vi "0036-Sub_WriteI2C.vi"(0 "device":T2, 1 "書き込み":u8[](array[numeric])=[2], 2 "numBytesToWrite":u8=1, 3 "error out":errorcluster) -> (7 "device 2":T2, 8 "数値":dbl, 10 "error out 2":errorcluster caption="error out")   [LabVIEW 2014]
uses:
  <userlib>/LV-CP2112_2014/LVProject/private/CP2112_device.ctl
  <userlib>/LV-CP2112_2014/LVProject/private/CP2112_SMBUS_S0.ctl
panel:
  out "numByteRead":u8
  out "HID_SMBUS_S0":T1
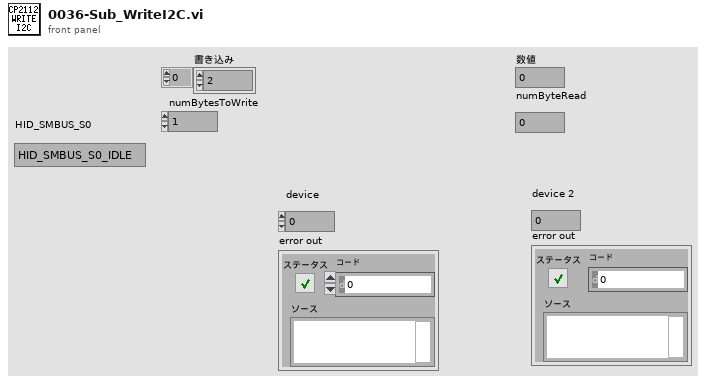
[diagram p1: front panel]
types:
  T1 = typedef "CP2112_SMBUS_S0.ctl" = enum8{"HID_SMBUS_S0_IDLE", "HID_SMBUS_S0_BUSY", "HID_SMBUS_S0_COMPLETE", "HID_SMBUS_S0_ERROR"}
  T2 = typedef "CP2112_device.ctl" = i32
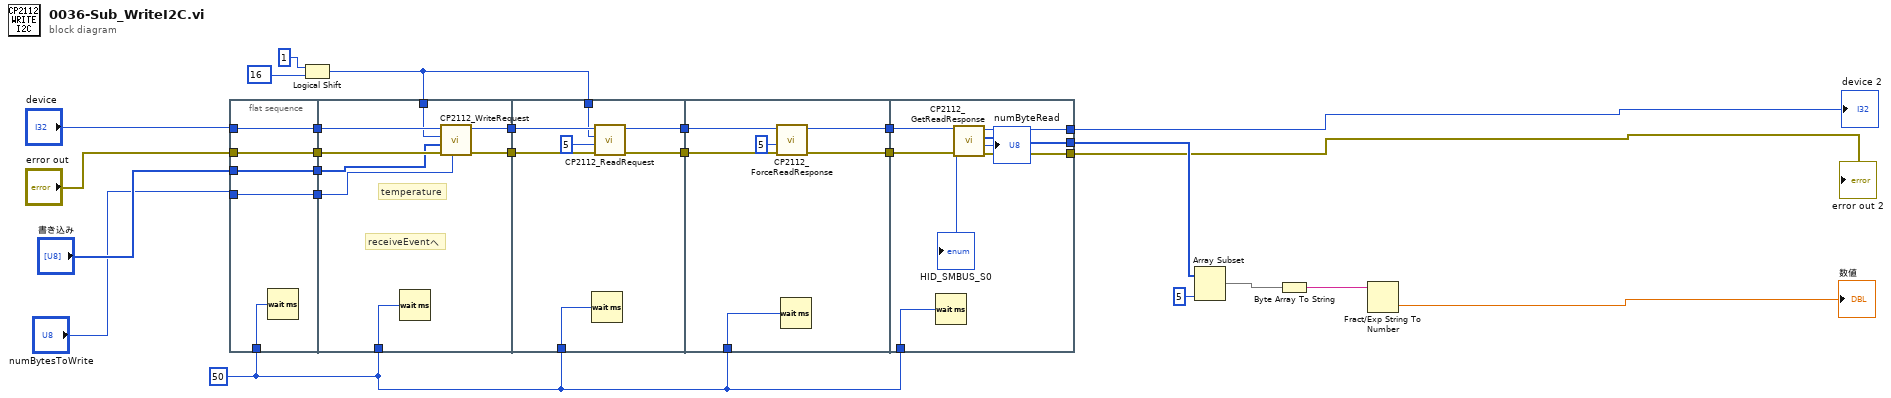
[diagram p0: block diagram]
diagram:
  w1 = u32 50 ("ミリ秒待機時間")
  n1 = flat-sequence {
    tunnel: "numBytesToWrite" -> [w27]
    tunnel: "書き込み" -> [w28]
    tunnel: "error out" -> [w29]
    tunnel: "device" -> [w30]
    tunnel: [w30] -> w5
    tunnel: [w29] -> w4
    tunnel: [w28] -> w3
    tunnel: [w27] -> w2
    tunnel: w1 -> [w26]
    tunnel: w16 -> [w34]
    tunnel: [w36] -> w25
    tunnel: [w35] -> w24
    tunnel: w1 -> [w33]
    tunnel: w5 -> [w38]
    tunnel: w4 -> [w37]
    tunnel: w3 -> [w32]
    tunnel: w2 -> [w31]
    tunnel: w25 -> [w41]
    tunnel: w24 -> [w42]
    tunnel: w16 -> [w40]
    tunnel: [w44] -> w23
    tunnel: [w43] -> w22
    tunnel: w1 -> [w39]
    tunnel: w23 -> [w49]
    tunnel: w22 -> [w48]
    tunnel: w1 -> [w47]
    tunnel: [w50] -> w21
    tunnel: [w51] -> w20
    tunnel: w21 -> [w55]
    tunnel: w20 -> [w54]
    tunnel: w1 -> [w53]
    tunnel: [w58] -> w9
    tunnel: [w57] -> w10
    tunnel: [w56] -> w15
    frame #0 {
      n2 = Wait (ms)(milliseconds to wait=w26) -> ()  [unwired: 1 out]
    }
    frame #1 {
      # "temperature"
      # "receiveEventへ"
      n3 = Wait (ms)(milliseconds to wait=w33) -> ()  [unwired: 1 out]
      n4 = call <userlib>:"CP2112_WriteRequest.vi"("numBytesToWrite"=w31, "error in (no error)"=w37, "buffer"=w32, "slaveAddress"=w34, "device"=w38) -> ("error out"=w36:errorcluster, "deviceOut"=w35:T2)  [unwired: 4 in, 1 out]
    }
    frame #2 {
      n5 = Wait (ms)(milliseconds to wait=w39) -> ()  [unwired: 1 out]
      n6 = call <userlib>:"CP2112_ReadRequest.vi"("error in (no error)"=w41, "numByteToRead"=i16 5, "slaveAddress"=w40, "device"=w42) -> ("error out"=w43:errorcluster, "deviceOut"=w44:T2)  [unwired: 5 in, 1 out]
    }
    frame #3 {
      n7 = call <userlib>:"CP2112_ForceReadResponse.vi"("error in (no error)"=w48, "numByteToRead"=i16 5, "device"=w49) -> ("error out"=w51:errorcluster, "deviceOut"=w50:T2)  [unwired: 6 in, 1 out]
      n8 = Wait (ms)(milliseconds to wait=w47) -> ()  [unwired: 1 out]
    }
    frame #4 {
      n9 = Wait (ms)(milliseconds to wait=w53) -> ()  [unwired: 1 out]
      n10 = call <userlib>:"CP2112_GetReadResponse.vi"("error in (no error)"=w54, "device"=w55) -> ("error out"=w58:errorcluster, "numByteRead"=→"numByteRead":u8, "buffer"=w56:u8[], "deviceOut"=w57:T2, "HID_SMBUS_S0"=→"HID_SMBUS_S0":T1)  [unwired: 4 in, 1 out]
    }
  }
  n11 = Logical Shift(y=1, x=16) -> (x << y=w16:i32)
  n12 = Array Subset(array=w15, length=5 ("長さ")) -> (w14:u8[])  [unwired: 1 in]
  n13 = Byte Array To String(unsigned byte array=w14) -> (string=w13:string)
  n14 = Fract/Exp String To Number(string=w13) -> (number=→"数値":dbl)  [unwired: 3 in, 1 out]
  "device 2" <- w10
  "error out 2" <- w9
